vi "Read ListItemObjects.vi"(8 "error in (no error)":errorcluster, 11 "AnalysisList in":refnum<class "AnalysisList.lvclass">) -> (0 "error out":errorcluster, 2 "AnalysisObjects":refnum<class "AnalysisListItems.lvclass">[](array[class]), 3 "AnalysisList out":refnum<class "AnalysisList.lvclass">)   [LabVIEW 2018, in "AnalysisList.lvclass"]
uses:
  AnalysisList.lvclass
  AnalysisListItems/AnalysisListItems.lvclass
  AnalysisList.lvclass/AnalysisList.ctl
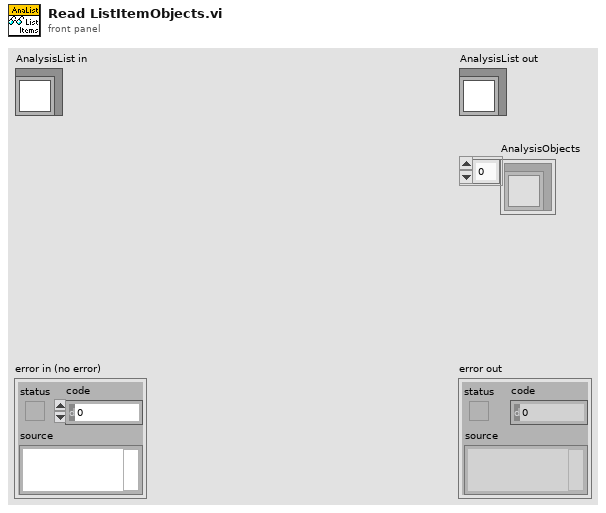
[diagram p1: front panel]
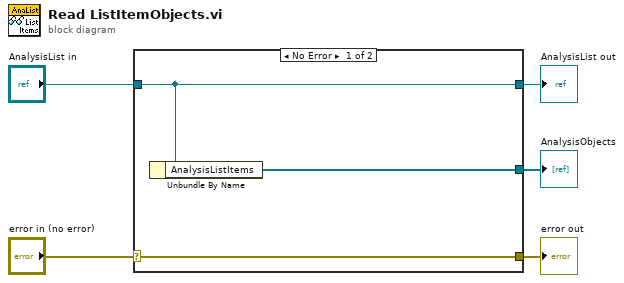
[diagram p0: block diagram]
diagram:
  n1 = case shown="No Error" "error in (no error)" {
    selector: "error in (no error)" -> [w8 w9]
    tunnel: [w8 w9] -> w4
    tunnel: [w7 w10] -> w2
    tunnel: "AnalysisList in" -> [w7 w10]
    tunnel: [w6 _] -> w1
    frame No Error {
      n2 = Unbundle By Name(w7) -> ("AnalysisListItems"=w6:refnum<class "AnalysisListItems.lvclass">[])
    }
    frame Error {
    }
  }
  "error out" <- w4
  "AnalysisList out" <- w2
  "AnalysisObjects" <- w1
